vi "test.vi"() -> ()   [LabVIEW 2020]
uses:
  typedefs/SSI_Init_Params.ctl
  typedefs/SSI_commands.ctl
panel:
  in  "Command args":string[](array[string])=["1", "2", "3"]
  in  "stop":bool
  out "return arguments":string[](array[string])
  in  "Initialization Parameters":T1
  in  "error in (no error)":errorcluster
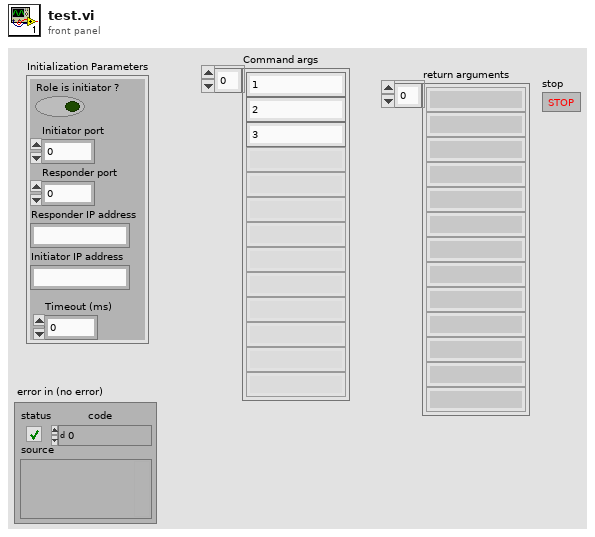
[diagram p1: front panel]
types:
  T1 = typedef "SSI_Init_Params.ctl" = cluster{"Role is initiator ?":bool, "Initiator port":i32, "Responder port":i32, "Responder IP address":string, "Initiator IP address":string, "Timeout (ms)":i32}
  T2 = typedef "SSI_commands.ctl" = enum16{"INIT", "ADD_COMMAND", "REMOVE_COMMAND", "QUERY", "SERVE"}
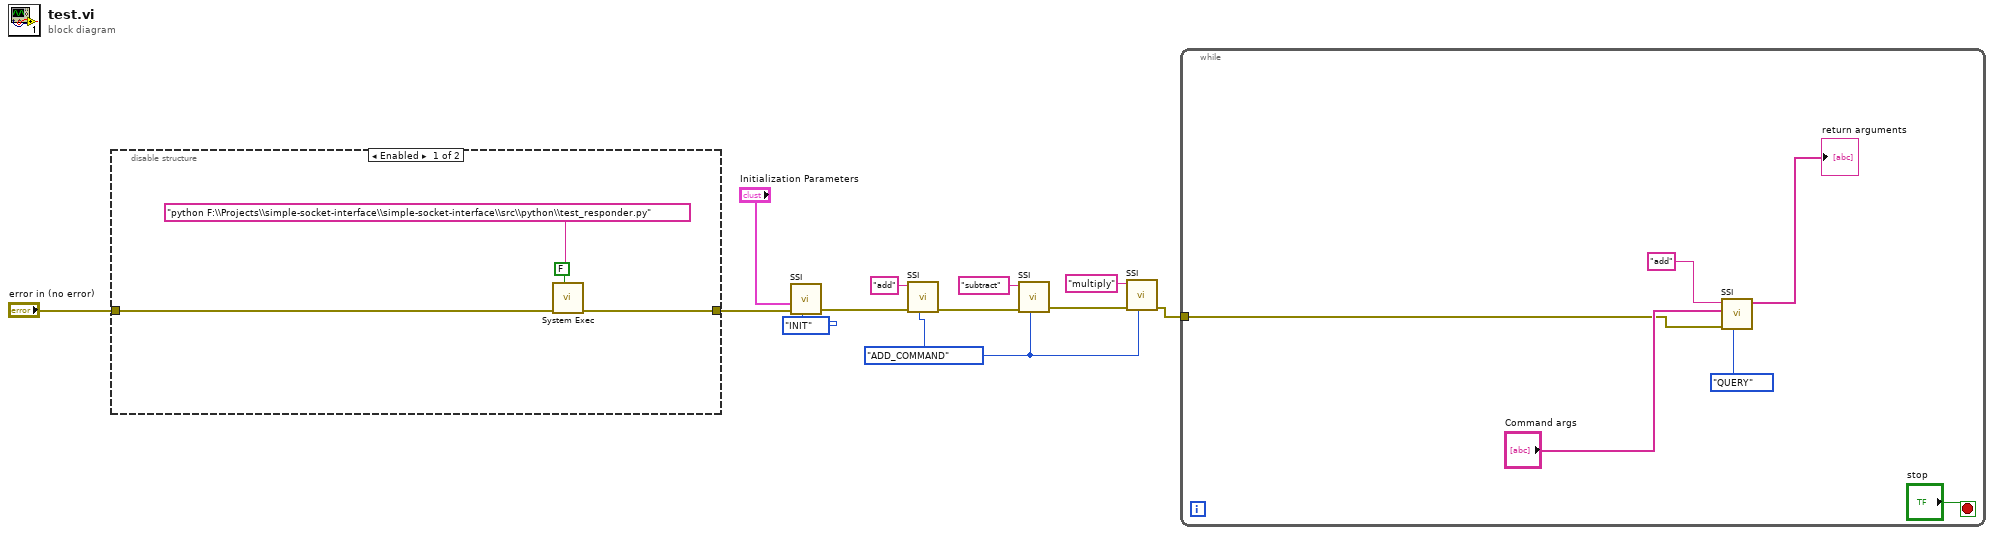
[diagram p0: block diagram]
diagram:
  w7 = SSI_commands."ADD_COMMAND" ("Command")
  n1 = disable-structure shown="Enabled" {
    disable-tunnel: "error in (no error)" -> [w15 w17]
    disable-tunnel: [w14 w17] -> w2
    frame Enabled {
      n2 = call <vilib>:"System Exec.vi"("wait until completion? (T)"=FALSE, "error in (no error)"=w15, "command line"="python F:\\Projects\\simple-socket-interface\\simple-socket-interface\\src\\python\\test_responder.py") -> ("error out"=w14:errorcluster)  [unwired: 5 in, 3 out]
    }
    frame Disabled {
    }
  }
  n3 = call "SSI.vi"("Command"=SSI_commands."INIT", "error in (no error)"=w2, "Initialization Parameters"="Initialization Parameters") -> ("error out"=w9:errorcluster)  [unwired: 7 in, 1 out]
  n4 = call "SSI.vi"("Command"=w7, "error in (no error)"=w9, "Command name"="add") -> ("error out"=w10:errorcluster)  [unwired: 7 in, 1 out]
  n5 = call "SSI.vi"("Command"=w7, "error in (no error)"=w10, "Command name"="subtract") -> ("error out"=w11:errorcluster)  [unwired: 7 in, 1 out]
  n6 = call "SSI.vi"("Command"=w7, "error in (no error)"=w11, "Command name"="multiply") -> ("error out"=w1:errorcluster)  [unwired: 7 in, 1 out]
  n7 = while {
    tunnel: w1 -> [w18]
    stop <- "stop" stop-if-true
    n8 = call "SSI.vi"("Command"=SSI_commands."QUERY", "error in (no error)"=w18, "Command args"="Command args", "Command name"="add") -> ("return arguments"=→"return arguments":string[])  [unwired: 6 in, 1 out]
  }
